vi "Player Info.vi"(8 "Victory Speech":string="All your base are belong to us!!", 9 "Name":string, 11 "Protector in":refnum<class "Protector.lvclass">) -> (3 "Protector out":refnum<class "Protector.lvclass">)   [LabVIEW 2015, in "Protector.lvclass"]
uses:
  Protector.lvclass
  Formics/Formics.lvclass
panel:
  # "Set default values for these two string controls"
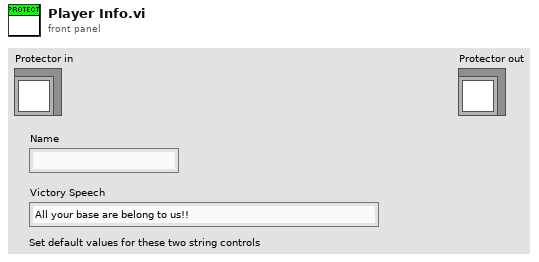
[diagram p1: front panel]
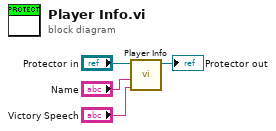
[diagram p0: block diagram]
diagram:
  n1 = call-parent "Player Info.vi"("Victory Speech"="Victory Speech", "Name"="Name", "Formics in"="Protector in") -> ("Formics out"=→"Protector out":refnum<class "Protector.lvclass">)  [unwired: 8 in]
